vi "Read Instr Addr.vi"(8 "error in (no error)":errorcluster, 11 "Power Supply Parent in":refnum<class "Power Supply Parent.lvclass">) -> (0 "error out":errorcluster, 2 "Instr Addr":refnum<visa-resource-name>, 3 "Power Supply Parent out":refnum<class "Power Supply Parent.lvclass">)   [LabVIEW 2017, in "Power Supply Driver.lvlib" / "Power Supply Parent.lvclass"]
uses:
  Power Supply Parent.lvclass
  Power Supply Parent.lvclass/Power Supply Parent.ctl
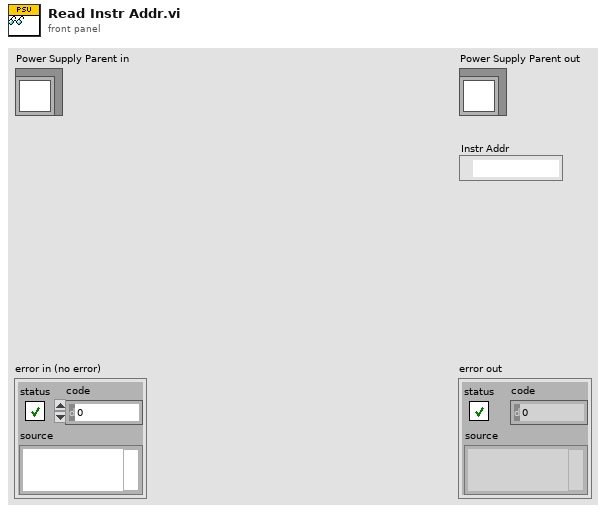
[diagram p1: front panel]
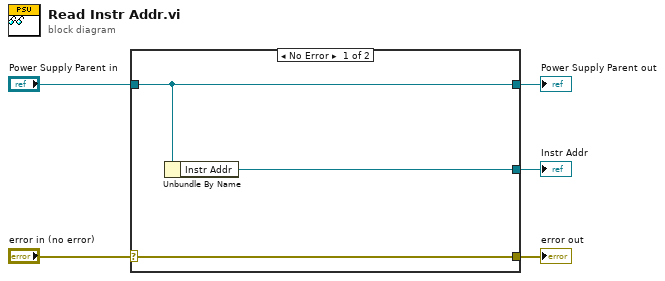
[diagram p0: block diagram]
diagram:
  n1 = case shown="No Error" "error in (no error)" {
    selector: "error in (no error)" -> [w8 w9]
    tunnel: [w8 w9] -> w4
    tunnel: [w7 w10] -> w2
    tunnel: "Power Supply Parent in" -> [w7 w10]
    tunnel: [w6 _] -> w1
    frame No Error {
      n2 = Unbundle By Name(w7) -> ("Instr Addr"=w6:refnum<visa-resource-name>)
    }
    frame Error {
    }
  }
  "error out" <- w4
  "Power Supply Parent out" <- w2
  "Instr Addr" <- w1
